vi "autonramp.vi"() -> ()   [LabVIEW 2012, in "Robohawks White.lvrbt"]
uses:
  Robohawks White.lvrbt
  <vilib>/NXT/Hardware/Plugins/Tetrix DC Motor/TetrixDCMotorAddress.ctl
  <vilib>/NXT/Block Support/NXT_InputPort.ctl
  <vilib>/NXT/Hardware/Plugins/Tetrix 180 deg Servo/Tetrix180ServoAddress.ctl
  <vilib>/NXT/NXTIO Xnodes/NXTIONodeSubVIs/TETRIX IO Check Battery.vi
  <vilib>/NXT/Dual Mode Library/Waits/Wait_Num(msec).vi
  <vilib>/NXT/NXTIO Xnodes/NXTIONodeSubVIs/TETRIX IO Stop DC Motors.vi
  <vilib>/NXT/Dual Mode Library/Waits/Wait_Num.vi
  <vilib>/NXT/NXTIO Xnodes/NXTIONodeSubVIs/TETRIX IO Move DC Motors.vi
  <vilib>/NXT/NXTIO Xnodes/NXTIONodeSubVIs/TETRIX IO Move Servos.vi
  <vilib>/NXT/Subs/LVHSConnector.ctl
  <vilib>/NXT/NXTIO Xnodes/AddressXNode/NXTIOAddress.xnode
  <vilib>/NXT/NXTIO Xnodes/NXTIOXNode/NXTIO.xnode
  <vilib>/NXT/LegoClasses/BrickReference/BrickReference.lvclass
panel:
  out "Enabled":bool
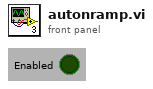
[diagram p1: front panel]
types:
  T1 = typedef "TetrixDCMotorAddress.ctl" = i32
  T2 = typedef "LVHSConnector.ctl" = refnum<class "BrickReference.lvclass">
  T3 = typedef "NXT_InputPort.ctl" = u32
  T4 = typedef "Tetrix180ServoAddress.ctl" = i32
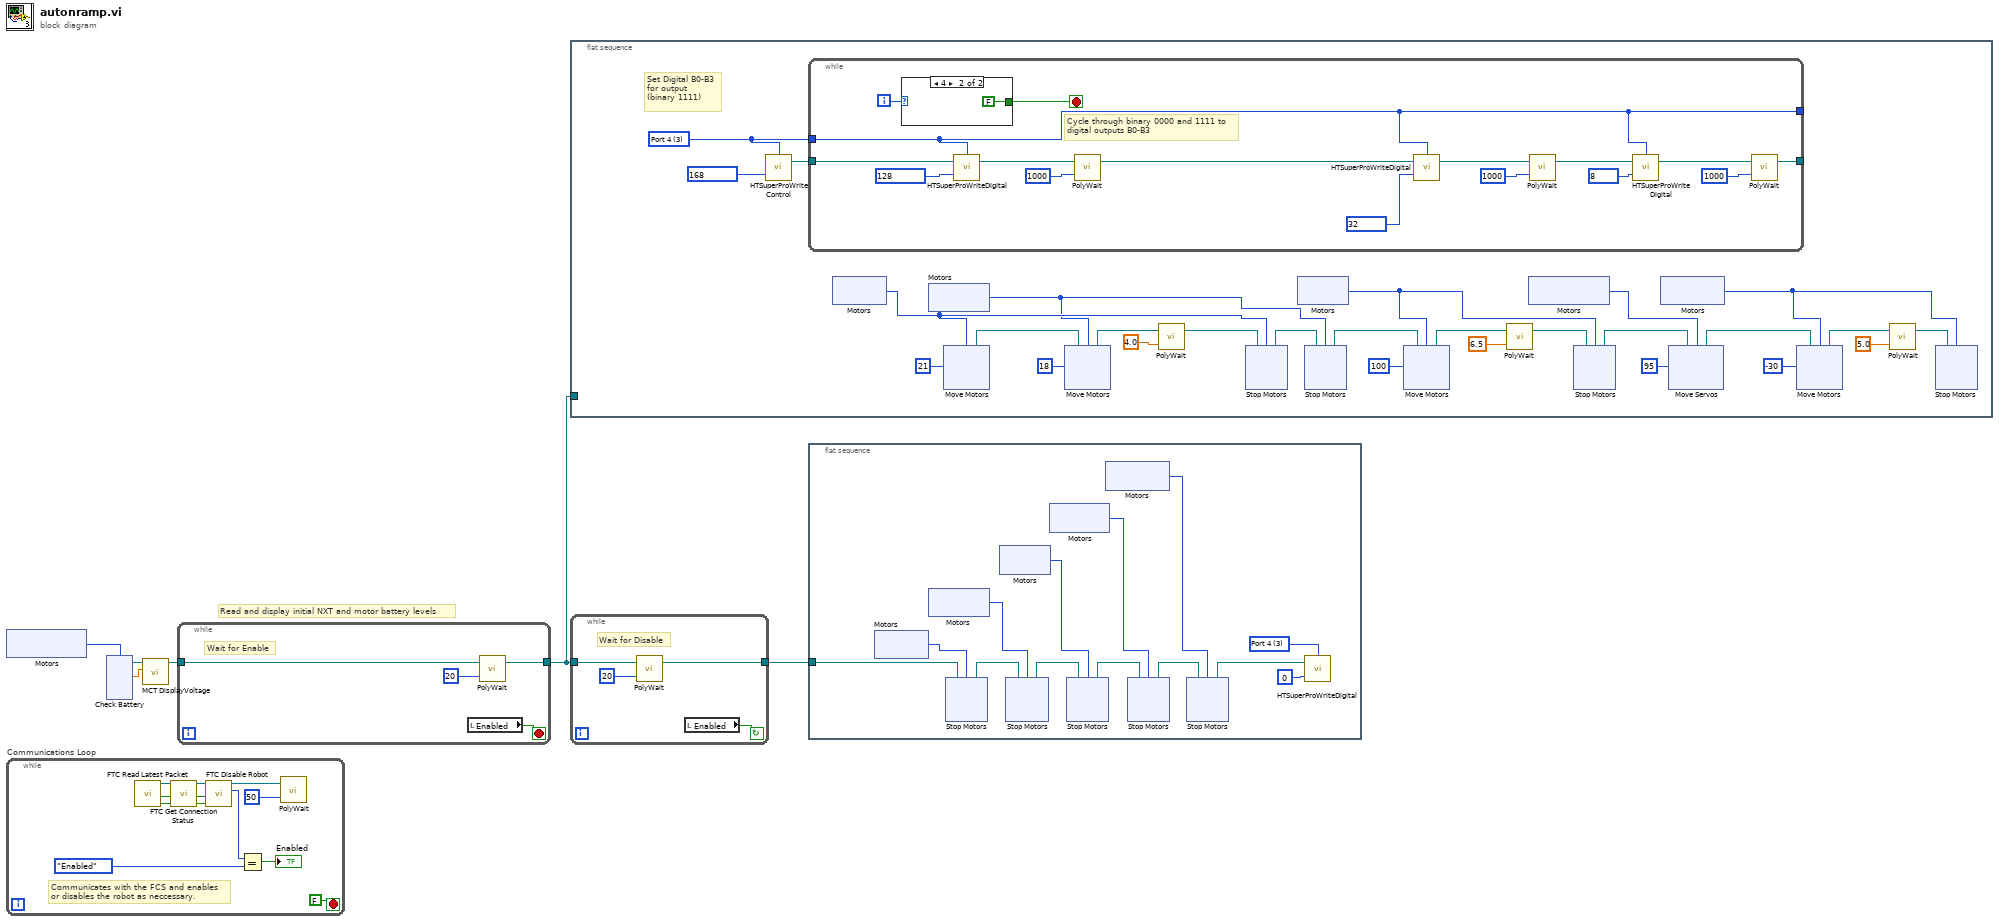
[diagram p0: block diagram]
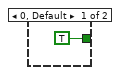
[diagram p2: hidden frame]
diagram:
  # "Read and display initial NXT and motor battery levels"
  n1 = xnode "Motors"() -> ("Motor"=w6:T1)
  n2 = while "Communications Loop" {
    stop <- FALSE stop-if-true
    # "Communicates with the FCS and enables \nor disables the robot as neccessary."
    n3 = call <vilib>:"FTC Read Latest Packet.vi"() -> ("Packet Received?"=w16:bool, "Stopped?"=w15:bool, "NXT/EV3"=w18:T2)  [unwired: 6 in, 3 out]
    n4 = call <vilib>:"FTC Get Connection Status.vi"("Packet Received?"=w16, "Stopped?"=w15, "NXT/EV3"=w18) -> ("Online?"=w7:bool, "Stopped?"=w8:bool, "NXT/EV3"=w17:T2)  [unwired: 5 in]
    n5 = call <vilib>:"FTC Disable Robot.vi"("Online?"=w7, "Stopped?"=w8, "NXT/EV3"=w17) -> ("Enabled?"=w11:enum16{"Disabled", "Enabled"}, "NXT/EV3"=w13:T2)  [unwired: 3 in]
    n6 = Equal?(x=w11, y=enum16{"Disabled", "Enabled"}."Enabled") -> (x = y?=→"Enabled":bool)
    n7 = call-poly <vilib>:"PolyWait.vi"("Time (100 msec)"=u32 50 ("Time (msec)"), "NXT/EV3"=w13) -> ()  [unwired: 2 in, 1 out]
  }
  n8 = xnode "Check Battery"("Motors"=w6) -> ("Voltage 1"=w1:sgl, "NXT/EV3"=w3:T2)  [unwired: 1 in]
  n9 = call <vilib>:"MCT DisplayVoltage.vi"("Motor Voltage"=w1, "NXT/EV3"=w3) -> ("NXT/EV3"=w2:T2)  [unwired: 9 in]
  n10 = while {
    tunnel: [w20] -> w5
    tunnel: w2 -> [w19]
    stop <- w21 stop-if-true
    # "Wait for Enable"
    n11 = local read "Enabled"() -> (w21:bool)
    n12 = call-poly <vilib>:"PolyWait.vi"("Time (100 msec)"=u32 20 ("Time (msec)"), "NXT/EV3"=w19) -> ("NXT/EV3"=w20:T2)  [unwired: 2 in]
  }
  n13 = flat-sequence {
    tunnel: w5 -> [_]
    frame #0 {
      w26 = T3 3 items=["Port 1", "Port 2", "Port 3", "Port 4"] ("Port")
      # "Set Digital B0-B3\nfor output\n(binary 1111)"
      n14 = call "HTSuperProWriteControl.vi"("Digital Control"=u8 168, "Port"=w26) -> ("NXT"=w25:T2)  [unwired: 3 in]
      n15 = while {
        tunnel: w25 -> [w65]
        tunnel: w26 -> [w50]
        tunnel: [w51] -> _
        tunnel: [w50] -> _
        i -> [w52]
        stop <- w53 stop-if-true
        # "Cycle through binary 0000 and 1111 to\ndigital outputs B0-B3"
        n16 = case shown="4" w52 {
          tunnel: [TRUE FALSE] -> w53
          frame 0, Default {
          }
          frame 4 {
          }
        }
        n17 = call "HTSuperProWriteDigital.vi"("Digital Value"=u8 128 ("Digital Control"), "NXT"=w65, "Port"=w50) -> ("NXT"=w63:T2)  [unwired: 2 in]
        n18 = call-poly <vilib>:"PolyWait.vi"("Time (100 msec)"=u32 1000, "NXT/EV3"=w63) -> ("NXT/EV3"=w58:T2)  [unwired: 2 in]
        n19 = call "HTSuperProWriteDigital.vi"("Digital Value"=u8 32 ("Digital Control"), "NXT"=w58, "Port"=w50) -> ("NXT"=w60:T2)  [unwired: 2 in]
        n20 = call-poly <vilib>:"PolyWait.vi"("Time (100 msec)"=u32 1000, "NXT/EV3"=w60) -> ("NXT/EV3"=w54:T2)  [unwired: 2 in]
        n21 = call "HTSuperProWriteDigital.vi"("Digital Value"=u8 8 ("Digital Control"), "NXT"=w54, "Port"=w50) -> ("NXT"=w56:T2)  [unwired: 2 in]
        n22 = call-poly <vilib>:"PolyWait.vi"("Time (100 msec)"=u32 1000, "NXT/EV3"=w56) -> ("NXT/EV3"=w51:T2)  [unwired: 2 in]
      }
      n23 = xnode "Motors"() -> ("Motor"=w45:T1)
      n24 = xnode "Motors"() -> ("Motor"=w44:T1)
      n25 = xnode "Move Motors"("Power/Speed 1"=i8 21, "Motors"=w45) -> ("NXT/EV3"=w49:T2)  [unwired: 1 in]
      n26 = xnode "Move Motors"("Power/Speed 1"=i8 18, "Motors"=w44, "NXT/EV3"=w49) -> ("NXT/EV3"=w23:T2)
      n27 = call-poly <vilib>:"PolyWait.vi"("Time (1 sec)"=sgl 4.0, "NXT/EV3"=w23) -> ("NXT/EV3"=w47:T2)  [unwired: 2 in]
      n28 = xnode "Stop Motors"("Motors"=w45, "NXT/EV3"=w47) -> ("NXT/EV3"=w46:T2)
      n29 = xnode "Motors"() -> ("Motor"=w39:T1)
      n30 = xnode "Stop Motors"("Motors"=w44, "NXT/EV3"=w46) -> ("NXT/EV3"=w43:T2)
      n31 = xnode "Move Motors"("Power/Speed 1"=i8 100, "Motors"=w39, "NXT/EV3"=w43) -> ("NXT/EV3"=w41:T2)
      n32 = call-poly <vilib>:"PolyWait.vi"("Time (1 sec)"=sgl 6.5, "NXT/EV3"=w41) -> ("NXT/EV3"=w40:T2)  [unwired: 2 in]
      n33 = xnode "Motors"() -> ("Motor"=w36:T4)
      n34 = xnode "Stop Motors"("Motors"=w39, "NXT/EV3"=w40) -> ("NXT/EV3"=w38:T2)
      n35 = xnode "Motors"() -> ("Motor"=w30:T1)
      n36 = xnode "Move Servos"("Position 1"=u8 95, "Motors"=w36, "NXT/EV3"=w38) -> ("NXT/EV3"=w34:T2)
      n37 = xnode "Move Motors"("Power/Speed 1"=i8 -30, "Motors"=w30, "NXT/EV3"=w34) -> ("NXT/EV3"=w32:T2)
      n38 = call-poly <vilib>:"PolyWait.vi"("Time (1 sec)"=sgl 5.0, "NXT/EV3"=w32) -> ("NXT/EV3"=w31:T2)  [unwired: 2 in]
      n39 = xnode "Stop Motors"("Motors"=w30, "NXT/EV3"=w31) -> ()  [unwired: 1 out]
    }
  }
  n40 = while {
    tunnel: [w129] -> w4
    tunnel: w5 -> [w128]
    stop <- w130 continue-if-true
    # "Wait for Disable"
    n41 = call-poly <vilib>:"PolyWait.vi"("Time (100 msec)"=u32 20 ("Time (msec)"), "NXT/EV3"=w128) -> ("NXT/EV3"=w129:T2)  [unwired: 2 in]
    n42 = local read "Enabled"() -> (w130:bool)
  }
  n43 = flat-sequence {
    tunnel: w4 -> [w144]
    frame #0 {
      w134 = T3 3 items=["Port 1", "Port 2", "Port 3", "Port 4"] ("Port")
      n44 = xnode "Motors"() -> ("Motor"=w143:T1)
      n45 = xnode "Motors"() -> ("Motor"=w142:T1)
      n46 = xnode "Stop Motors"("Motors"=w143, "NXT/EV3"=w144) -> ("NXT/EV3"=w140:T2)
      n47 = xnode "Motors"() -> ("Motor"=w141:T1)
      n48 = xnode "Stop Motors"("Motors"=w142, "NXT/EV3"=w140) -> ("NXT/EV3"=w139:T2)
      n49 = xnode "Motors"() -> ("Motor"=w138:T1)
      n50 = xnode "Stop Motors"("Motors"=w141, "NXT/EV3"=w139) -> ("NXT/EV3"=w137:T2)
      n51 = xnode "Motors"() -> ("Motor"=w136:T1)
      n52 = xnode "Stop Motors"("Motors"=w138, "NXT/EV3"=w137) -> ("NXT/EV3"=w135:T2)
      n53 = xnode "Stop Motors"("Motors"=w136, "NXT/EV3"=w135) -> ("NXT/EV3"=w133:T2)
      n54 = call "HTSuperProWriteDigital.vi"("Digital Value"=u8 0 ("Digital Control"), "NXT"=w133, "Port"=w134) -> ()  [unwired: 2 in, 1 out]
    }
  }
